vi "crio.vi"() -> ()   [LabVIEW 2019]
uses:
  <resource>/objmgr/ni.dex.rc
panel:
  in  "stop":bool
  out "Is Connected":bool
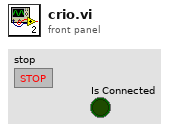
[diagram p1: front panel]
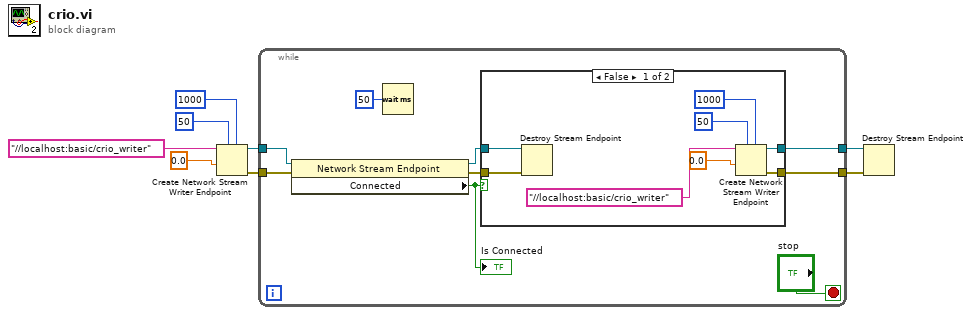
[diagram p0: block diagram]
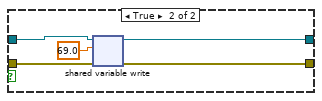
[diagram p2: hidden frame]
diagram:
  n1 = Create Network Stream Writer Endpoint(5:1000 ("timeout in ms (-1)"), 7:50 ("writer buffer size"), 9:0.0, 11:"//localhost:basic/crio_writer" ("writer name")) -> (0:w3:errorcluster, 3:w4:refnum<k21>)  [unwired: 3 in]
  n2 = while {
    tunnel: [w15] -> w2
    tunnel: [w14] -> w1
    tunnel: w4 -> [w12]
    tunnel: w3 -> [w11]
    stop <- "stop" stop-if-true
    n3 = property class="Network Stream Endpoint"(reference=w12, error in=w11) -> (reference out=w17:refnum<k21>, error out=w16:errorcluster, "Connected"=w13:bool)
    "Is Connected" <- w13
    n4 = Wait (ms)(milliseconds to wait=u32 50) -> ()  [unwired: 1 out]
    n5 = case shown="False" w13 {
      tunnel: w17 -> [w19 w28]
      tunnel: w16 -> [w20 w27]
      tunnel: [w22 w30] -> w15
      tunnel: [w21 w29] -> w14
      frame False {
        n6 = Destroy Stream Endpoint(8:w20, 11:w19) -> ()  [unwired: 1 out]
        n7 = Create Network Stream Writer Endpoint(5:1000 ("timeout in ms (-1)"), 7:50 ("writer buffer size"), 9:0.0, 11:"//localhost:basic/crio_writer" ("writer name")) -> (0:w21:errorcluster, 3:w22:refnum<k21>)  [unwired: 3 in]
      }
      frame True {
        n8 = shared-variable-write(w28, w27, 69.0) -> (w30:refnum<k21>, w29:errorcluster)  [unwired: 1 in, 1 out]
      }
    }
  }
  n9 = Destroy Stream Endpoint(8:w1, 11:w2) -> ()  [unwired: 1 out]
